vi "normalise Y.vi"(6 "Y-axis absolute":bool, 9 "Country index":u16, 10 "Populations":i64[](array[numeric]), 11 "Y in":i32[](array[numeric])) -> (3 "Y out":dbl[](array[numeric]))   [LabVIEW 2019]
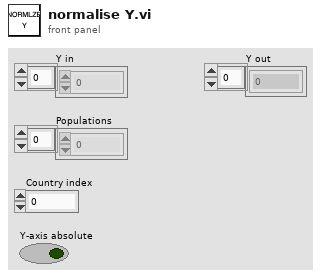
[diagram p1: front panel]
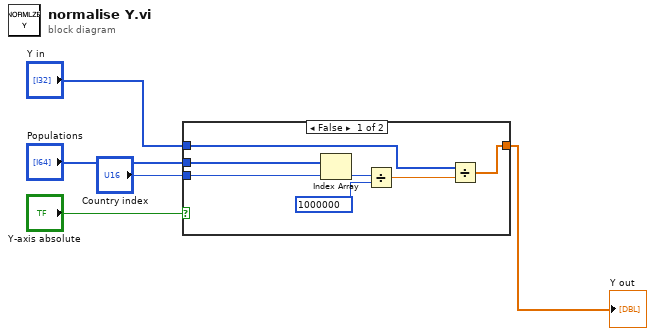
[diagram p0: block diagram]
diagram:
  n1 = case shown="False" "Y-axis absolute" {
    tunnel: "Populations" -> [w12 _]
    tunnel: "Y in" -> [w8 w13]
    tunnel: [w7 w13] -> w3
    tunnel: "Country index" -> [w6 _]
    frame False {
      n2 = Index Array(array=w12, index=w6) -> (element=w11:i64)
      n3 = Divide(x=w11, y=i64 1000000) -> (x/y=w9:dbl)
      n4 = Divide(x=w8, y=w9) -> (x/y=w7:dbl[])
    }
    frame True {
    }
  }
  "Y out" <- w3
